vi "PMUParseConfigUnits.vi"(10 "PMUConfig":T1 {"DigitalStatusMask" format="%b"; "Valid Inputs" format="%b"}, 11 "PacketBody":u8[](array[numeric])) -> (2 "PMUConfig":T1 {"DigitalStatusMask" format="%b"; "Valid Inputs" format="%b"}, 3 "PacketBody":u8[](array[numeric]))   [LabVIEW 2014, in "SensorPlugins.lvlib" / "C37.118 PMU.lvclass"]
uses:
  C37.118 PMU.lvclass
  Typedef/PMUConfigData.ctl
  Typedef/FormatBits.ctl
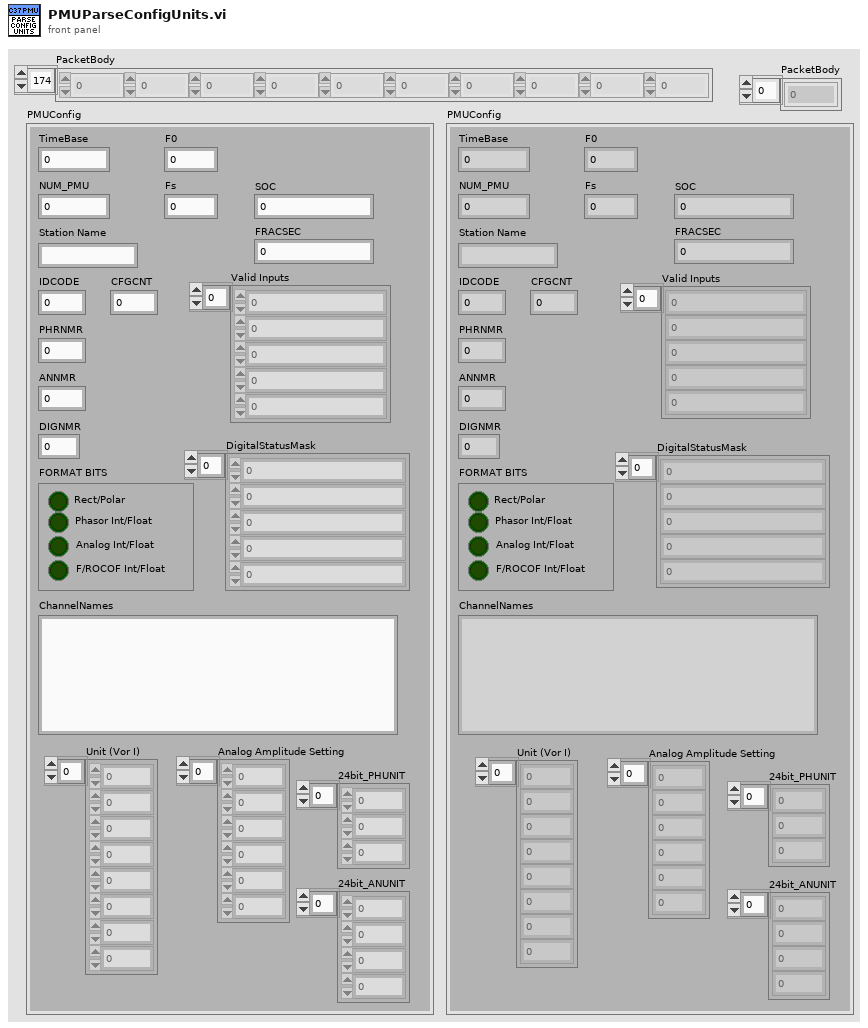
[diagram p1: front panel]
types:
  T1 = typedef "SensorPlugins.lvlib/C37.118 PMU.lvclass/PMUConfigData.ctl" = cluster{"TimeBase":u32, "NUM_PMU":u16, "Station Name":string, "IDCODE":u16, "PHRNMR":u16, "ANNMR":u16, "DIGNMR":u16, "FORMAT BITS":T2, "Valid Inputs":u16[], "DigitalStatusMask":u16[], "24bit_PHUNIT":i32[], "24bit_ANUNIT":u32[], "Analog Amplitude Setting":u32[], "Unit (Vor I)":u8[], "ChannelNames":string, "Fs":i16, "SOC ":u32, "FRACSEC":u32, "F0":sgl, "CFGCNT":u16}
  T2 = typedef "SensorPlugins.lvlib/C37.118 PMU.lvclass/FormatBits.ctl" = cluster{"Rect/Polar":bool, "Phasor Int/Float":bool, "Analog Int/Float":bool, "F/ROCOF Int/Float":bool}
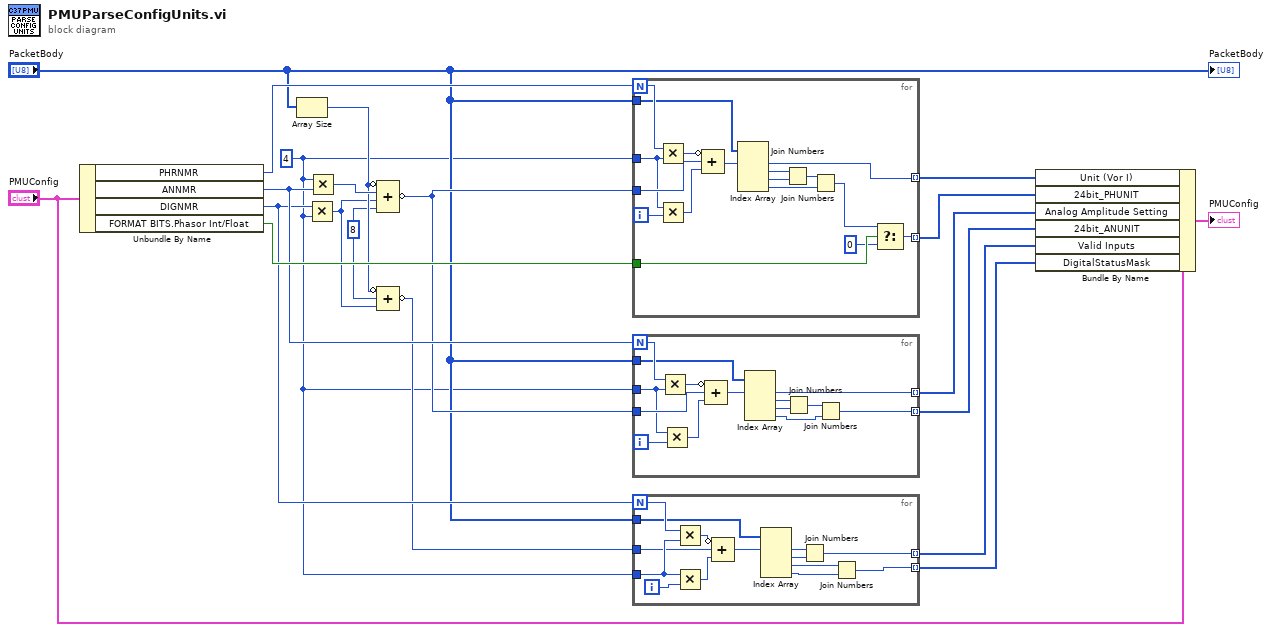
[diagram p0: block diagram]
diagram:
  w8 = 8 ("value")
  w1 = u16 4 ("y")
  n1 = Unbundle By Name("PMUConfig") -> ("PHRNMR"=w20:u16, "ANNMR"=w14:u16, "DIGNMR"=w10:u16, "FORMAT BITS.Phasor Int/Float"=w19:bool)
  n2 = Array Size(array="PacketBody") -> (size(s)=w9:i32)
  n3 = Multiply(x=w10, y=w1) -> (x*y=w7:u16)
  n4 = Multiply(x=w1, y=w14) -> (x*y=w15:u16)
  n5 = Compound Arithmetic op=ADD(invert w9, w15, w7, w8) -> (invert w13:i32)
  n6 = Compound Arithmetic op=ADD(invert w9, w8, w7) -> (invert w6:i32)
  n7 = for {
    N: w20 -> [w37]
    tunnel: "PacketBody" -> [w28]
    tunnel: w19 -> [w23]
    tunnel: [w24] -> w16 mode=indexing
    tunnel: [w29] -> w17 mode=indexing
    tunnel: w1 -> [w25]
    tunnel: w13 -> [w26]
    i -> [w35]
    n8 = Multiply(x=w37, y=w25) -> (x*y=w36:i32)
    n9 = Multiply(x=w25, y=w35) -> (x*y=w27:i32)
    n10 = Compound Arithmetic op=ADD(invert w36, w26, w27) -> (w34:i32)
    n11 = Index Array(array=w28, index #1=w34) -> (element #1=w29:u8, element #2=w33:u8, element #3=w32:u8, element #4=w30:u8)  [unwired: 3 in]
    n12 = Join Numbers(hi=w33, lo=w32) -> ((hi.lo)=w31:u16)
    n13 = Join Numbers(hi=w31, lo=w30) -> ((hi.lo)=w22:u32)
    n14 = Select(t=w22, s=w23, f=u32 0 ("t")) -> (s? t:f=w24:u32)
  }
  n15 = for {
    N: w14 -> [w51]
    tunnel: w1 -> [w48]
    tunnel: w13 -> [w49]
    tunnel: "PacketBody" -> [w44]
    tunnel: [w43] -> w12 mode=indexing
    tunnel: [w38] -> w11 mode=indexing
    i -> [w47]
    n16 = Multiply(x=w51, y=w48) -> (x*y=w50:i32)
    n17 = Multiply(x=w48, y=w47) -> (x*y=w46:i32)
    n18 = Compound Arithmetic op=ADD(invert w50, w49, w46) -> (w45:i32)
    n19 = Index Array(array=w44, index #1=w45) -> (element #1=w43:u8, element #2=w42:u8, element #3=w41:u8, element #4=w39:u8)  [unwired: 3 in]
    n20 = Join Numbers(hi=w42, lo=w41) -> ((hi.lo)=w40:u16)
    n21 = Join Numbers(hi=w40, lo=w39) -> ((hi.lo)=w38:u32)
  }
  n22 = for {
    N: w10 -> [w65]
    tunnel: "PacketBody" -> [w58]
    tunnel: w1 -> [w64]
    tunnel: w6 -> [w63]
    tunnel: [w53] -> w5 mode=indexing
    tunnel: [w56] -> w4 mode=indexing
    i -> [w60]
    n23 = Multiply(x=w65, y=w64) -> (x*y=w62:i32)
    n24 = Multiply(x=w64, y=w60) -> (x*y=w61:i32)
    n25 = Compound Arithmetic op=ADD(invert w62, w63, w61) -> (w59:i32)
    n26 = Index Array(array=w58, index #1=w59) -> (element #1=w55:u8, element #2=w54:u8, element #3=w52:u8, element #4=w57:u8)  [unwired: 3 in]
    n27 = Join Numbers(hi=w55, lo=w54) -> ((hi.lo)=w53:u16)
    n28 = Join Numbers(hi=w52, lo=w57) -> ((hi.lo)=w56:u16)
  }
  n29 = Bundle By Name(cluster="PMUConfig", "Unit (Vor I)"=w17, "24bit_PHUNIT"=w16, "Analog Amplitude Setting"=w12, "24bit_ANUNIT"=w11, "Valid Inputs"=w5, "DigitalStatusMask"=w4) -> (→"PMUConfig":T1)
  "PacketBody" <- "PacketBody"
